vi "Register Remote Messages.vi"(8 "error in (no error)":errorcluster, 9 "Types":string[](array[string]), 10 "EnQr":refnum<class "Message Enqueuer.lvclass">, 11 "RemoteMessaging in":refnum<class "RemoteMessaging.lvclass">) -> (0 "error out":errorcluster, 3 "RemoteMessaging out":refnum<class "RemoteMessaging.lvclass">)   [LabVIEW 2020, in "Volatus.lvlib" / "RemoteMessaging.lvclass"]
uses:
  RemoteMessaging.lvclass
  RemoteMessaging.lvclass/RemoteMessaging.ctl
  <vilib>/Utility/miscctls.llb/LVMapReplaceAction.ctl
  <vilib>/ActorFramework/Message Enqueuer/Message Enqueuer.lvclass
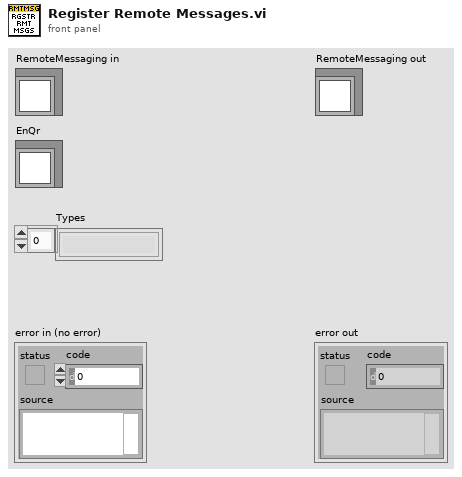
[diagram p1: front panel]
types:
  T1 = typedef "LVMapReplaceAction.ctl" = enum32{"Modify Entry only if found", "Add or Modify Entry", "Delete Entry"}
  T2 = map{string, refnum<class "Message Enqueuer.lvclass">[]}
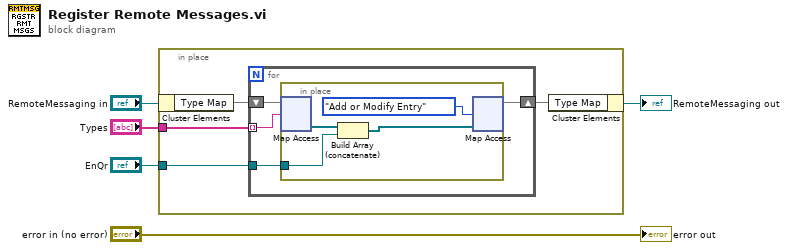
[diagram p0: block diagram]
diagram:
  n1 = in-place {
    in-place-border: "Types" -> [w7]
    in-place-border: "EnQr" -> [w6]
    n2 = in-place-cluster #1("RemoteMessaging in") -> ("Type Map"=w9:T2)
    n3 = for {
      shift-right: [w10] -> w8
      shift-left: w9 -> [w13]
      tunnel: w7 -> [w12] mode=indexing
      tunnel: w6 -> [w11]
      n4 = in-place {
        in-place-border: w11 -> [w16]
        n5 = in-place-map #2(w13, w12) -> (w17:refnum<class "Message Enqueuer.lvclass">[])  [unwired: 1 in, 1 out]
        n6 = Build Array (concatenate)(w17, w16) -> (w15:refnum<class "Message Enqueuer.lvclass">[])
        n7 = in-place-map #2(w15, LVMapReplaceAction."Add or Modify Entry" ("action")) -> (w10:T2)  [unwired: 2 out]
      }
    }
    n8 = in-place-cluster #1("Type Map"=w8) -> (→"RemoteMessaging out":refnum<class "RemoteMessaging.lvclass">)
  }
  "error out" <- "error in (no error)"
